vi "Convert CI PWM Module to Slot Configuration.vi"(8 "error in":errorcluster, 9 "module":refnum<class "Module.lvclass">, 10 "RSI module":refnum<class "RSI Module.lvclass">, 11 "slot ref in":T1 format="%.0x") -> (0 "error out":errorcluster, 3 "slot ref out":T1 format="%.0x")   [LabVIEW 2020, in "Scan Engine Scripting.lvlib"]
uses:
  Scan Engine Scripting.lvlib
  <vilib>/NI VeriStand/Custom Device API/Custom Device Item Ref.ctl
  Modules.lvlibp/RSI Module/RSI Module.lvclass
  Modules/Module/Module.lvclass
  Modules.lvlibp/SD Module/SD Module.lvclass
  C:/jenkins/workspace/ercat-custom-device_release_20.4/Custom Device Source/Modules.lvlibp/RSI Module/RSI Module.lvclass
  Modules.lvlibp/SD Module/Type Defs/Counter.ctl
  Modules.lvlibp/SD Module/Type Defs/Counter Channel.ctl
  Modules.lvlibp/SD Module/Type Defs/Count Edges.ctl
  Modules.lvlibp/SD Module/Type Defs/Period Measurement.ctl
  Modules.lvlibp/SD Module/Type Defs/Pulse Width Measurement.ctl
  Modules.lvlibp/SD Module/Type Defs/Frequency Measurement.ctl
  Modules/Mode Classes/Controls/SD DIO Mode.ctl
  Modules/Mode Classes/Controls/SD Measurement Mode.ctl
  <vilib>/NI VeriStand/Custom Device API/Custom Device API.lvlib
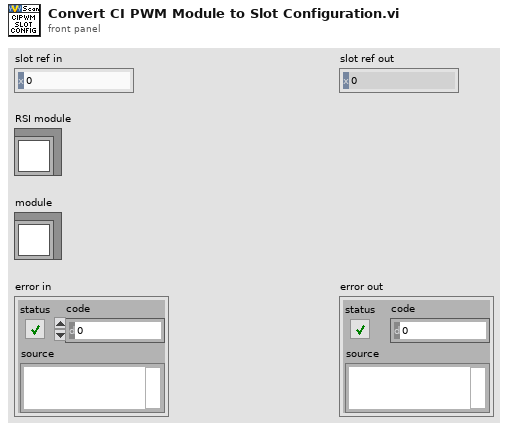
[diagram p1: front panel]
types:
  T1 = typedef "Custom Device API.lvlib/Custom Device Item Ref.ctl" = u64
  T2 = typedef "Scan Engine Scripting.lvlib/SD DIO Mode.ctl" = u32
  T3 = typedef "Modules.lvlibp/SD Module.lvclass/Counter Channel.ctl" = cluster{"Measurement Mode":u32, "Count Edges":T4, "Period Measurement":T5, "Pulse Width Measurement":T6, "Frequency Measurement":T7}
  T4 = typedef "Modules.lvlibp/SD Module.lvclass/Count Edges.ctl" = cluster{"Counter Event":u32, "Counter Source":u32, "Counter Direction":u32, "Terminal Count":u32, "Output Mode":u32, "Gate Mode":u32}
  T5 = typedef "Modules.lvlibp/SD Module.lvclass/Period Measurement.ctl" = cluster{"Measurement Edge":u32}
  T6 = typedef "Modules.lvlibp/SD Module.lvclass/Pulse Width Measurement.ctl" = cluster{"Measurement Type":u32}
  T7 = typedef "Modules.lvlibp/SD Module.lvclass/Frequency Measurement.ctl" = cluster{"Measurement Edge":u32, "Measurement Timebase":u32}
  T8 = typedef "Modules.lvlibp/SD Module.lvclass/Counter.ctl" = cluster{"Counter Channels":T3[]}
  T9 = typedef "Scan Engine Scripting.lvlib/counter input pwm channel settings.ctl" = cluster{"name":string, "default value":dbl, "measurement type":T10}
  T10 = typedef "Scan Engine Scripting.lvlib/PWM Input Channel.lvclass/Measurement Type.ctl" = enum16{"High Pulse", "Low Pulse", "Most Recent"}
  T11 = typedef "Scan Engine Scripting.lvlib/SD Measurement Mode.ctl" = u32
  T12 = typedef "Modules.lvlibp/Custom Device API.lvlib/Custom Device Item Ref.ctl" = u64
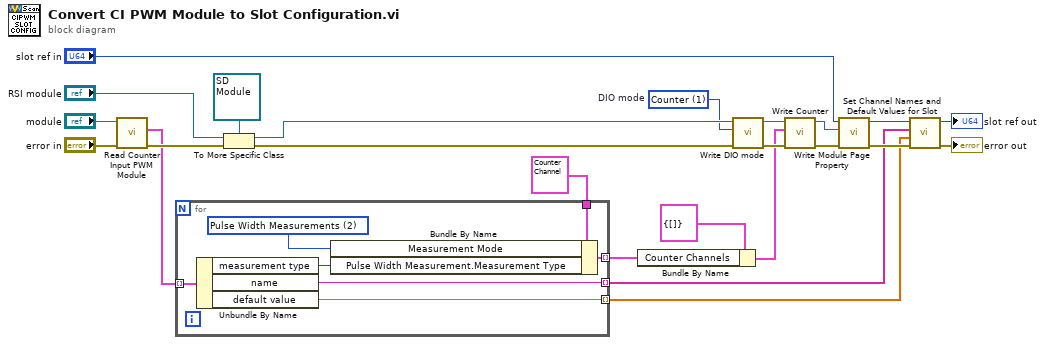
[diagram p0: block diagram]
diagram:
  w1 = T2 1 items=["Normal", "Counter", "Counter Slave", "PWM", "Quadrature"]  # DIO mode
  n1 = call-dynamic "Read Counter Input PWM Module.vi"("error in"="error in", "module in"="module") -> ("error out"=w16:errorcluster, "channel settings"=w4:T9[])  [unwired: 7 in, 1 out]
  n2 = for {
    tunnel: T3 {"Measurement Mode"=2, "Count Edges"={"Counter Event"=0, "Counter Source"=0, "Counter Direction"=0, "Terminal Count"=4294967295, "Output Mode"=0, "Gate Mode"=3}, "Period Measurement"={"Measurement Edge"=0}, "Pulse Width Measurement"={"Measurement Type"=3}, "Frequency Measurement"={"Measurement Edge"=0, "Measurement Timebase"=0}} ("Counter Channel") -> [w31]
    tunnel: [w30] -> w5 mode=indexing
    tunnel: w4 -> [w29] mode=indexing
    tunnel: [w27] -> w3 mode=indexing
    tunnel: [w26] -> w2 mode=indexing
    w25 = T11 2 items=["Count Edges", "Period Measurements", "Pulse Width Measurements", "Frequency Measurements"] ("Measurement Mode")
    n3 = Unbundle By Name(w29) -> ("measurement type"=w28:T10, "name"=w27:string, "default value"=w26:dbl)
    n4 = Bundle By Name(cluster=w31, "Measurement Mode"=w25, "Pulse Width Measurement.Measurement Type"=w28) -> (w30:T3)
  }
  n5 = To More Specific Class(target class=refnum<class "SD Module.lvclass"> refnum ("Modules.lvlibp:SD Module.lvclass"), reference="RSI module", error in=w16) -> (specific class reference=w18:refnum<class "SD Module.lvclass">, error out=w20:errorcluster)
  n6 = Bundle By Name(cluster=T8 {"Counter Channels"=[]} ("Counter"), "Counter Channels"=w5) -> (w6:T8)
  n7 = call-dynamic "Write DIO mode.vi"("error in (no error)"=w20, "DIO mode"=w1, "SD Module in"=w18) -> ("error out"=w10:errorcluster, "SD Module out"=w9:refnum<class "SD Module.lvclass">)  [unwired: 7 in]
  n8 = call-dynamic "Write Counter.vi"("error in (no error)"=w10, "Counter"=w6, "SD Module in"=w9) -> ("error out"=w7:errorcluster, "SD Module out"=w8:refnum<class "SD Module.lvclass">)  [unwired: 7 in]
  n9 = call "Write Module Page Property.vi"("error in (no error)"=w7, "RSI Module"=w8, "Node Ptr In"="slot ref in") -> ("error out"=w21:errorcluster, "Node Ptr Out"=w22:T12)  [unwired: 6 in, 1 out]
  n10 = call "Set Channel Names and Default Values for Slot.vi"("error in"=w21, "default values"=w2, "channel names"=w3, "slot ref in"=w22) -> ("error out"=→"error out":errorcluster, "slot ref out"=→"slot ref out":T1)  [unwired: 6 in]
